vi "Read Values.vi"(8 "error in (no error)":errorcluster, 11 "Scope in":refnum<class "Scope.lvclass">) -> (0 "error out":errorcluster, 2 "Values":dbl[](array[numeric]), 3 "Scope out":refnum<class "Scope.lvclass">)   [LabVIEW 2020, in "Scope.lvlib" / "Scope.lvclass"]
uses:
  Scope.lvclass
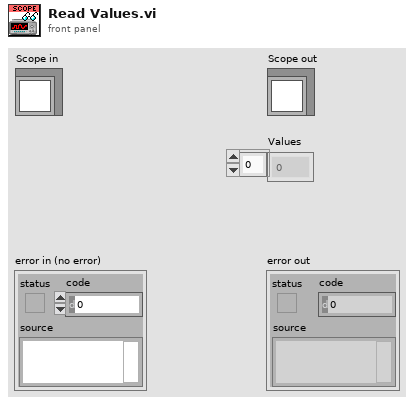
[diagram p1: front panel]
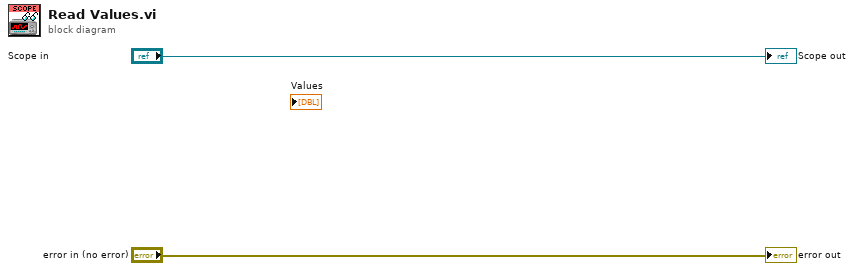
[diagram p0: block diagram]
diagram:
  "error out" <- "error in (no error)"
  "Scope out" <- "Scope in"
